vi "Analog Write N Chans.vi"(7 "Analog Ref Override":dbl, 8 "Error In":errorcluster, 9 "AO Values":dbl[](array[numeric]), 10 "AO Channel(s)":u8[](array[numeric]), 11 "LINX Resource":T1) -> (0 "Error Out":errorcluster, 3 "LINX Resource":T1)   [LabVIEW 2019, in "LMH-LINX.lvlib"]
doc: "Write value(s) to the specified analog output channel(s)."
uses:
  <vilib>/MakerHub/LINX/LMH-LINX.lvlib
  <vilib>/MakerHub/LINX/Private/Type Defs/LINX Ref.ctl
  <vilib>/MakerHub/LINX/Private/Type Defs/Platform.ctl
  <vilib>/MakerHub/LINX/Private/Type Defs/Interface.ctl
  <vilib>/MakerHub/LINX/Private/Device/Type Defs/LINX Device Config.ctl
  <vilib>/MakerHub/LINX/Private/Device/Type Defs/TCP Config.ctl
  <vilib>/MakerHub/LINX/Private/Device/Type Defs/Channels.ctl
  <vilib>/MakerHub/LINX/Private/Type Defs/Peripheral.ctl
  <vilib>/MakerHub/LINX/Private/Type Defs/Error Type.ctl
  <vilib>/MakerHub/LINX/Private/myRIO/myRIO.lvlib
  <vilib>/MakerHub/LINX/Private/Device/Device.lvlib
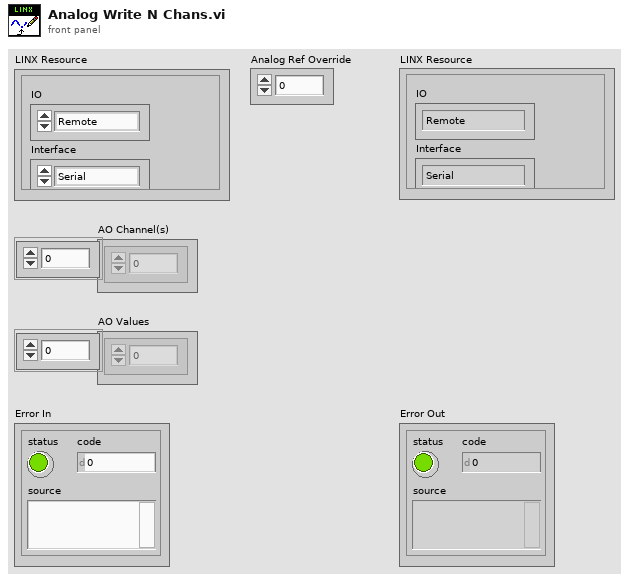
[diagram p1: front panel]
types:
  T1 = typedef "LMH-LINX.lvlib/LINX Ref.ctl" = cluster{"IO":T2, "Interface":T3, "LINX Device Config":T4}
  T2 = typedef "LMH-LINX.lvlib/Platform.ctl" = enum16{"Remote", "Local"}
  T3 = typedef "LMH-LINX.lvlib/Interface.ctl" = enum16{"Serial", "TCP"}
  T4 = typedef "LMH-LINX.lvlib/Device.lvlib/LINX Device Config.ctl" = cluster{"Interface":T3, "COM Port":refnum<visa-resource-name>, "TCP Configuration":T5, "Device Family":u8, "Device ID":u8, "Device Name":string, "TCP Ref":refnum<k5>, "Channels":T6}
  T5 = typedef "LMH-LINX.lvlib/Device.lvlib/TCP Config.ctl" = cluster{"IP Address":string, "Port":u16}
  T6 = typedef "LMH-LINX.lvlib/Channels.ctl" = cluster{"DI":u8[], "DO":u8[], "AI":u8[], "AO":u8[], "PWM":u8[], "QE":u8[], "UART":u8[], "I2C 2":u8[], "SPI":u8[], "CAN":u8[], "Servo":u8[], "AI Ref (V)":dbl, "AI Resolution (Bits)":u8, "AO Ref (V)":dbl, "AO Resolution (Bits)":u8}
  T7 = typedef "LMH-LINX.lvlib/Peripheral.ctl" = enum8{"DI", "DO", "AI", "AO", "PWM", "QE", "UART", "I2C", "SPI", "CAN", "Servo"}
  T8 = typedef "LMH-LINX.lvlib/Error Type.ctl" = enum16{"Unknown", "Timeout", "Corrupt Return Packet", "Unable To Connect", "Command Not Supported", "Channel DNE", "Invalid COM Config", "Firmware Version Mismatch", "myRIO Support", "CMD Specific Error", "Local IO Not Supported"}
  T9 = typedef "AO.lvlib/AO Reference.ctl" = cluster{"myRIO Reference":T10, "AO Channel List":T14, "AO Scaling Constant List":T16}
  T10 = typedef "myRIO Generic Hardware Reference.ctl" = cluster{"myRIO Model":T11, "myRIO Hardware Reference":T12}
  T11 = typedef "Hardware Version Enum.ctl" = enum16{"Unknown", "myRIO-1900", "myRIO-1950"}
  T12 = typedef "myRIO v1.0 Reference.ctl" = cluster{"Generic FPGA Reference":T13, "Allow multiple opens":bool}
  T13 = typedef "Generic FPGA Reference.ctl" = refnum<k20>
  T14 = typedef "AO Channels List.ctl" = T15[]
  T15 = typedef "AO Channels Enum.ctl" = enum16{"Not Connected", "AudioOut/Left", "AudioOut/Right", "C/AO0", "C/AO1", "A/AO0", "A/AO1", "B/AO0", "B/AO1"}
  T16 = typedef "Analog Scaling Constants List.ctl" = T17[]
  T17 = typedef "Analog Scaling Constants.ctl" = cluster{"LSB Weight (Volts)":dbl, "Offset (Volts)":dbl, "Signed?":bool}
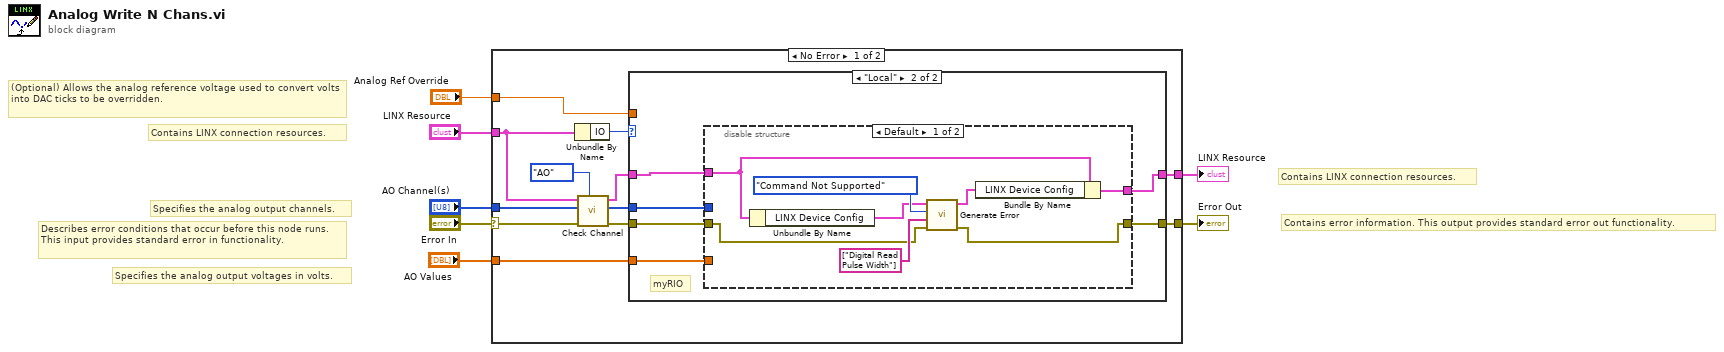
[diagram p0: block diagram]
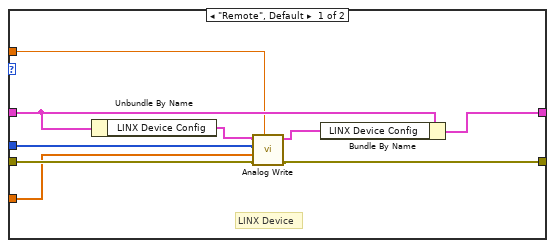
[diagram p2: hidden frame]
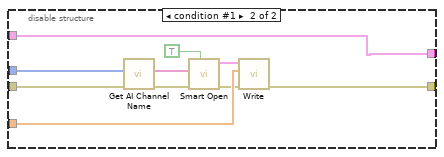
[diagram p3: hidden frame]
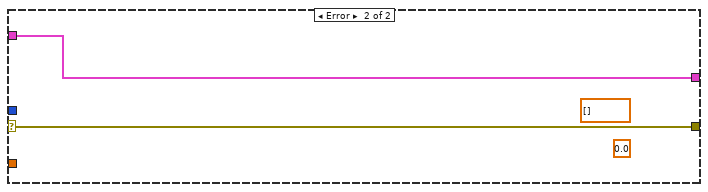
[diagram p4: hidden frame]
diagram:
  # "Contains LINX connection resources."
  # "Contains error information. This output provides standard error out functionality."
  # "Specifies the analog output voltages in volts."
  # "Specifies the analog output channels."
  # "(Optional) Allows the analog reference voltage used to convert volts into DAC ticks to be overridden."
  # "Contains LINX connection resources."
  # "Describes error conditions that occur before this node runs. This input provides standard error in functionality."
  n1 = case shown="No Error" "Error In" {
    selector: "Error In" -> [w9 w54]
    tunnel: [w18 w54] -> w7
    tunnel: [w17 w53] -> w6
    tunnel: "LINX Resource" -> [w12 w53]
    tunnel: "AO Channel(s)" -> [w11 _]
    tunnel: "Analog Ref Override" -> [w10 _]
    tunnel: "AO Values" -> [w8 _]
    frame No Error {
      n2 = Unbundle By Name(w12) -> ("IO"=w19:T2)
      n3 = call <vilib>:"Check Channel.vi"("Peripheral"=Peripheral."AO", "Error In"=w9, "Channels"=w11, "LINX Resource"=w12) -> ("Error Out"=w16:errorcluster, "Channels"=w15:u8[], "LINX Resource"=w13:T1)  [unwired: 5 in]
      n4 = case shown="\"Local\"" w19 {
        tunnel: w16 -> [w23 w32]
        tunnel: w13 -> [w28 w29]
        tunnel: [w24 w33] -> w18
        tunnel: [w27 w30] -> w17
        tunnel: w15 -> [w22 w34]
        tunnel: w10 -> [w20 _]
        tunnel: w8 -> [w21 w31]
        frame "Remote", Default {
          # "LINX Device"
          n5 = Unbundle By Name(w28) -> ("LINX Device Config"=w26:T4)
          n6 = call <vilib>:"Analog Write.vi"("Analog Ref Override"=w20, "Error In"=w23, "AO Values"=w21, "AO Channels"=w22, "LINX Device Config"=w26) -> ("Error Out"=w24:errorcluster, "LINX Device Config"=w25:T4)  [unwired: 5 in]
          n7 = Bundle By Name(cluster=w28, "LINX Device Config"=w25) -> (w27:T1)
        }
        frame "Local" {
          # "myRIO"
          n8 = disable-structure shown="Default" {
            disable-tunnel: w34 -> [_ w52]
            disable-tunnel: [w38 w51] -> w33
            disable-tunnel: w32 -> [w37 w49]
            disable-tunnel: w31 -> [_ w47]
            disable-tunnel: w29 -> [w36 w43]
            disable-tunnel: [w35 w43] -> w30
            frame condition #0 (active) {
              n9 = Unbundle By Name(w36) -> ("LINX Device Config"=w41:T4)
              n10 = call <vilib>:"Generate Error.vi"("Error In"=w37, "Arguments"=string[] ["Digital Read Pulse Width"], "Error Type"=Error_Type."Command Not Supported", "LINX Device Config"=w41) -> ("Error Out"=w38:errorcluster, "Dup LINX Device Config"=w40:T4)  [unwired: 6 in]
              n11 = Bundle By Name(cluster=w36, "LINX Device Config"=w40) -> (w35:T1)
            }
            frame condition #1 {
              n12 = call <vilib>:"Get AI Channel Name.vi"("Error In"=w49, "AI Channel Nums"=w52) -> ("Error Out"=w48:errorcluster, "AI Channels"=w50:string[])  [unwired: 7 in]
              n13 = call <vilib>:"Smart Open.vi"("Allow multiple opens?"=TRUE, "error in (no error)"=w48, "Channel Names"=w50) -> ("error out"=w45:errorcluster, "AO Ref Out"=w46:T9)  [unwired: 7 in]
              n14 = call <vilib>:"Write.vi"("error in (no error)"=w45, "Values"=w47, "AO Ref In"=w46) -> ("error out"=w51:errorcluster)  [unwired: 6 in, 1 out]
            }
          }
        }
      }
    }
    frame Error {
      (unwired) 0.0 ("AI Ref")
      (unwired) dbl[] [] ("Values")
    }
  }
  "Error Out" <- w7
  "LINX Resource" <- w6
